vi "TeleopMatchInfo.vi"(10 "Call Context":T2, 11 "Match Info":T1={"Autonomous Elapsed Seconds"=0.0, "TeleOp Elapsed Seconds"=0.0, "Disabled Elapsed Seconds"=0.0, "Visited Autonomous"=FALSE, "Visited TeleOp"=FALSE, "Visited Disabled"=FALSE, "Autonomous Settings"={"Autonomous Style"=enum."Independent", "VI Refnum"=refnum}}) -> ()   [LabVIEW 2018]
uses:
  <vilib>/Rock Robotics/WPI/DriverStation/WPI_DriverStationDerivedRobotMode.ctl
  <vilib>/Rock Robotics/WPI/DriverStation/WPI_DriverStationMatch Info.ctl
  <userlib>/836-Library/System/TDMS_V2/Support/TDMS_DevRef.ctl
  <userlib>/836-Library/System/TDMS_V2/Support/Logging_Settings.ctl
  <userlib>/836-Library/System/TDMS_V2/Support/Group_FIFO_Config.ctl
  <userlib>/836-Library/System/TDMS_V2/Support/Channel_FIFO_Config.ctl
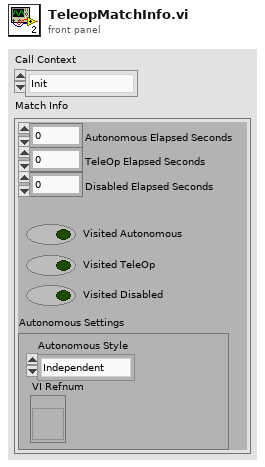
[diagram p1: front panel]
types:
  T1 = typedef "WPI_DriverStationMatch Info.ctl" = cluster{"Autonomous Elapsed Seconds":dbl, "TeleOp Elapsed Seconds":dbl, "Disabled Elapsed Seconds":dbl, "Visited Autonomous":bool, "Visited TeleOp":bool, "Visited Disabled":bool, "Autonomous Settings":cluster{"Autonomous Style":enum16{"Iterative", "Independent"}, "VI Refnum":refnum<vi>}}
  T2 = typedef "WPI_DriverStationDerivedRobotMode.ctl" = enum16{"Init", "Execute", "Stop"}
  T3 = typedef "TDMS_DevRef.ctl" = cluster{"Name":string, "File Ref":refnum<k34>, "Start Time":timestamp, "Logging Settings":T4, "Group FIFO Config":T5[], "Data To Write":refnum<data-value>, "semaphore":T7, "Ref Time Reset":refnum<k4>}
  T4 = typedef "Logging_Settings.ctl" = cluster{"Data Grab Period":dbl, "File Write Period":dbl, "Max Stored Size":dbl, "Burst Size":dbl}
  T5 = typedef "Group_FIFO_Config.ctl" = cluster{"Group":string, "Channels":T6[], "Channel Names":string[]}
  T6 = typedef "Channel_FIFO_Config.ctl" = cluster{"Channel":string, "FIFO":refnum<k33>}
  T7 = typedef "Semaphore RefNum" = refnum<k1>
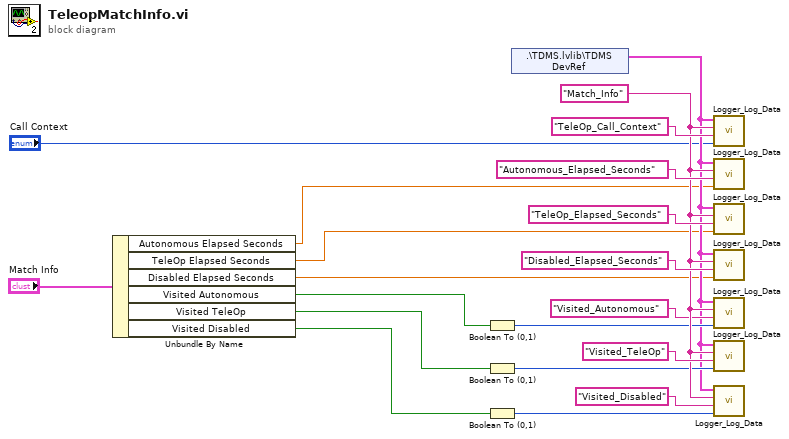
[diagram p0: block diagram]
diagram:
  w13 = "Match_Info" ("Group")
  n1 = Unbundle By Name("Match Info") -> ("Autonomous Elapsed Seconds"=w6:dbl, "TeleOp Elapsed Seconds"=w5:dbl, "Disabled Elapsed Seconds"=w4:dbl, "Visited Autonomous"=w3:bool, "Visited TeleOp"=w2:bool, "Visited Disabled"=w1:bool)
  n2 = Boolean To (0,1)(Boolean=w3) -> (0, 1=w11:i16)
  n3 = Boolean To (0,1)(Boolean=w2) -> (0, 1=w10:i16)
  n4 = Boolean To (0,1)(Boolean=w1) -> (0, 1=w9:i16)
  n5 = shared-variable ".\\TDMS.lvlib\\TDMS DevRef"() -> (w8:T3)  [unwired: 1 in, 1 out]
  n6 = call <userlib>:"Logger_Log_Data.vi"("Data"="Call Context", "Channel"="TeleOp_Call_Context", "Group"=w13, "TDMS DevRef"=w8) -> ()  [unwired: 7 in, 1 out]
  n7 = call <userlib>:"Logger_Log_Data.vi"("Data"=w6, "Channel"="Autonomous_Elapsed_Seconds", "Group"=w13, "TDMS DevRef"=w8) -> ()  [unwired: 7 in, 1 out]
  n8 = call <userlib>:"Logger_Log_Data.vi"("Data"=w5, "Channel"="TeleOp_Elapsed_Seconds", "Group"=w13, "TDMS DevRef"=w8) -> ()  [unwired: 7 in, 1 out]
  n9 = call <userlib>:"Logger_Log_Data.vi"("Data"=w4, "Channel"="Disabled_Elapsed_Seconds", "Group"=w13, "TDMS DevRef"=w8) -> ()  [unwired: 7 in, 1 out]
  n10 = call <userlib>:"Logger_Log_Data.vi"("Data"=w11, "Channel"="Visited_Autonomous", "Group"=w13, "TDMS DevRef"=w8) -> ()  [unwired: 7 in, 1 out]
  n11 = call <userlib>:"Logger_Log_Data.vi"("Data"=w10, "Channel"="Visited_TeleOp", "Group"=w13, "TDMS DevRef"=w8) -> ()  [unwired: 7 in, 1 out]
  n12 = call <userlib>:"Logger_Log_Data.vi"("Data"=w9, "Channel"="Visited_Disabled", "Group"=w13, "TDMS DevRef"=w8) -> ()  [unwired: 7 in, 1 out]
